vi "Test_freq_generator_5160.vi"() -> ()   [LabVIEW 2013]
uses:
  <vilib>/measure/maspectr.llb/Power Spectrum and PSD Export Mode.ctl
  <vilib>/measure/maspectr.llb/FFT Power Spectrum and PSD for 1 Chan (CDB).vi
  <vilib>/measure/NI_MAPro.lvlib
panel:
  out "power spectrum":cluster{"f0":dbl, "df":dbl, "magnitude":dbl[]}(graph)
  out "Cos":fxp<+/-,16,0>[](array[numeric])
  out "simdata":i16[](array[numeric])
  out "Sin":fxp<+/-,16,0>[](array[numeric])
  out "Waveform Graph 2":i16[](graph)
  out "Waveform Graph":dbl[][](graph)
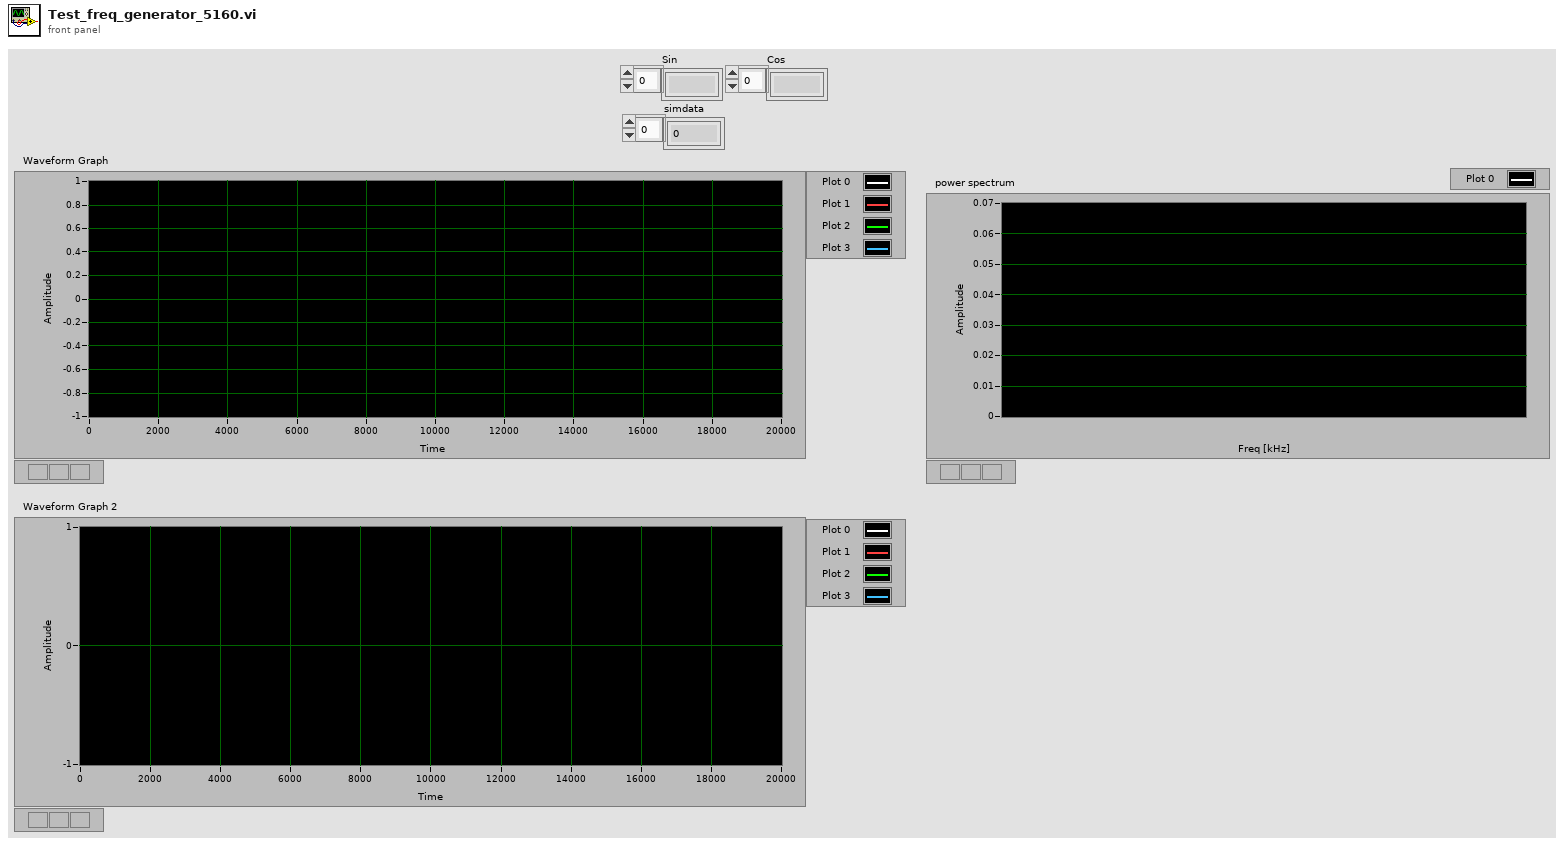
[diagram p1: front panel]
types:
  T1 = typedef "NI_MAPro.lvlib/Power Spectrum and PSD Export Mode.ctl" = u16
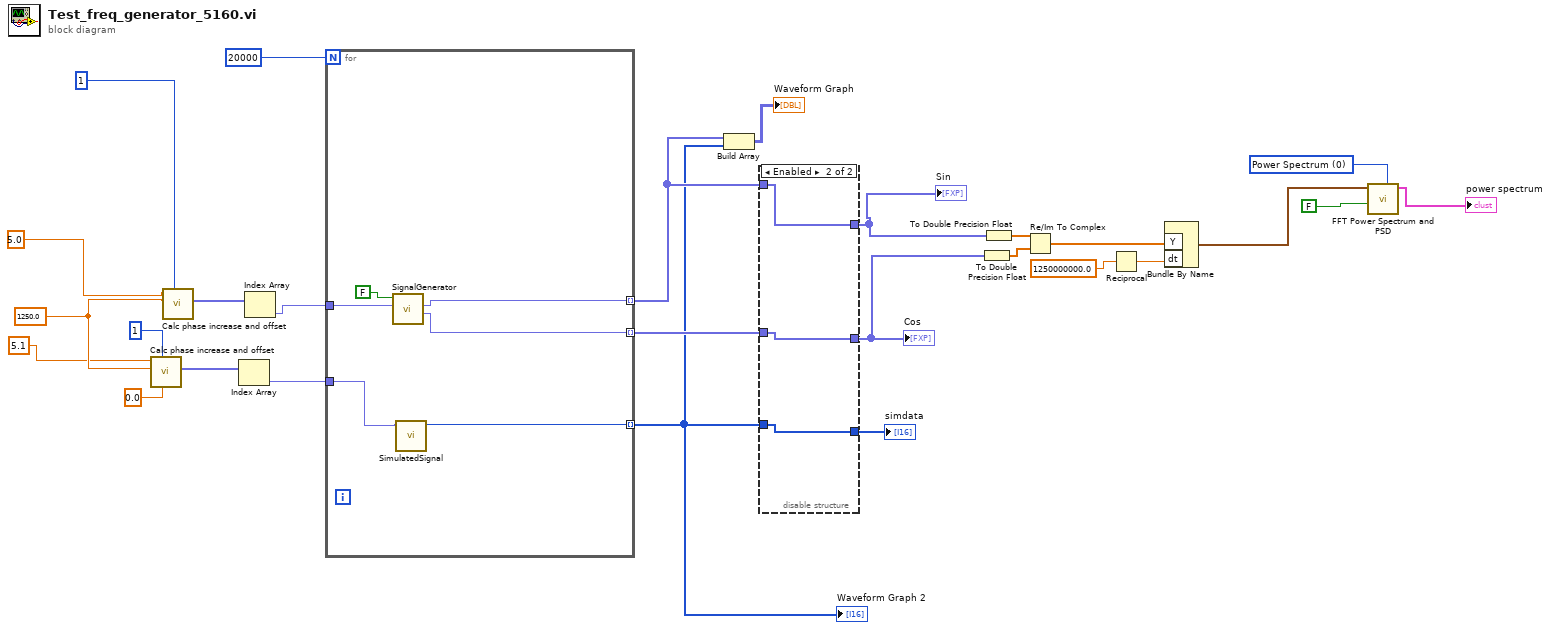
[diagram p0: block diagram]
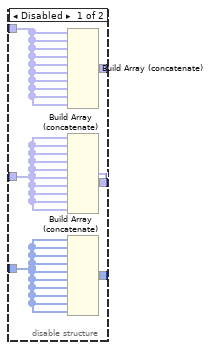
[diagram p2: hidden frame]
diagram:
  w15 = T1 0 items=["Power Spectrum", "Power Spectral Density"] ("export mode")
  w22 = 1250.0 ("fclk (800MHz)")
  n1 = call "Calc phase increase and offset.vi"("Phase offset (deg)"=0.0, "# of DDS"=1, "fclk (MHz)"=w22, "f_generated (MHz)"=5.1) -> ("Phase out"=w18:fxp<+,64,64>[])  [unwired: 5 in, 2 out]
  n2 = call "Calc phase increase and offset.vi"("# of DDS"=1, "fclk (MHz)"=w22, "f_generated (MHz)"=5.0) -> ("Phase out"=w20:fxp<+,64,64>[])  [unwired: 6 in, 2 out]
  n3 = Index Array(array=w18) -> (element=w17:fxp<+,64,64>)  [unwired: 1 in]
  n4 = Index Array(array=w20) -> (element=w19:fxp<+,64,64>)  [unwired: 1 in]
  n5 = for {
    N: 20000 -> [_]
    tunnel: w19 -> [w33]
    tunnel: [w30] -> w4 mode=indexing
    tunnel: w17 -> [w31]
    tunnel: [w29] -> w2 mode=indexing
    tunnel: [w28] -> w16 mode=indexing
    n6 = call "SignalGenerator.vi"("phase"=w33, "Reset"=FALSE ("reset")) -> ("Cos"=w28:fxp<+/-,16,0>, "Sin"=w30:fxp<+/-,16,0>)  [unwired: 7 in, 1 out]
    n7 = call "SimulatedSignal.vi"("phase"=w31) -> ("Sample output"=w29:i16)  [unwired: 9 in, 1 out]
  }
  "Waveform Graph 2" <- w2
  n8 = Build Array(w4, w2) -> (→"Waveform Graph":fxp<+/-,32,16>[][])
  n9 = disable-structure shown="Enabled" {
    disable-tunnel: w16 -> [w39 w41]
    disable-tunnel: [w38 w42] -> w6
    disable-tunnel: [w37 w41] -> w5
    disable-tunnel: w4 -> [w36 w42]
    disable-tunnel: w2 -> [w35 w40]
    disable-tunnel: [w34 w40] -> w1
    frame Disabled {
      n10 = Build Array (concatenate)(w36, w36, w36, w36, w36, w36, w36, w36, w36, w36) -> (w38:fxp<+/-,16,0>[])
      n11 = Build Array (concatenate)(w39, w39, w39, w39, w39, w39, w39, w39, w39, w39) -> (w37:fxp<+/-,16,0>[])
      n12 = Build Array (concatenate)(w35, w35, w35, w35, w35, w35, w35, w35, w35, w35) -> (w34:i16[])
    }
    frame Enabled {
    }
  }
  "Sin" <- w6
  "simdata" <- w1
  "Cos" <- w5
  n13 = To Double Precision Float(number=w5) -> (double precision float=w8:dbl[])
  n14 = To Double Precision Float(number=w6) -> (double precision float=w9:dbl[])
  n15 = Re/Im To Complex(1:w8, 2:w9) -> (0:w7:cdb[])
  n16 = Reciprocal(x=1250000000.0 ("dt")) -> (1/x=w11:dbl)
  n17 = Bundle By Name("Y"=w7, "dt"=w11) -> (w14:waveform(cdb))  [unwired: 1 in]
  n18 = call-poly <vilib>:"FFT Power Spectrum and PSD.vi"("export mode"=w15, "dB On (F)"=FALSE, "time signal"=w14) -> ("Power Spectrum / PSD"=→"power spectrum":cluster{"f0":dbl, "df":dbl, "magnitude":dbl[]})  [unwired: 5 in, 3 out]
